vi "Hex string to byte array.vi"(8 "Error In":errorcluster, 11 "Hex string":string) -> (0 "Error Out":errorcluster, 3 "Byte Array":u8[](array[numeric]) format="%02x")   [LabVIEW 2020]
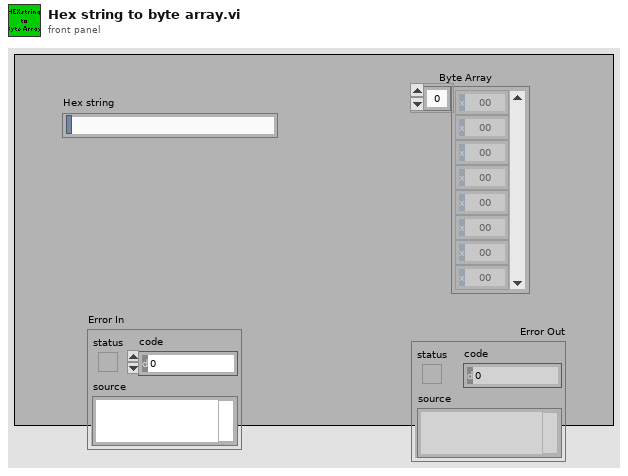
[diagram p1: front panel]
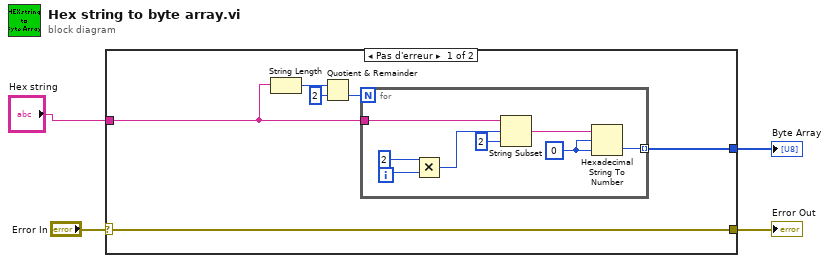
[diagram p0: block diagram]
diagram:
  n1 = case shown="Pas d'erreur" "Error In" {
    selector: "Error In" -> [w10 w19]
    tunnel: [w10 w19] -> w3
    tunnel: "Hex string" -> [w6 _]
    tunnel: [w5 _] -> w2
    frame No Error {
      n2 = String Length(string=w6) -> (length=w7:i32)
      n3 = Quotient & Remainder(x=w7, y=2) -> (floor(x/y)=w9:i32)  [unwired: 1 out]
      n4 = for {
        N: w9 -> [_]
        tunnel: w6 -> [w18]
        tunnel: [w11] -> w5 mode=indexing
        i -> [w17]
        w12 = u8 0 ("default (0 U32)")
        n5 = Multiply(x=2, y=w17) -> (x*y=w15:i32)
        n6 = String Subset(string=w18, offset (0)=w15, length (rest)=2 ("length (rest)")) -> (substring=w13:string)
        n7 = Hexadecimal String To Number(string=w13, offset=w12, default (0uL)=w12) -> (number=w11:u8)  [unwired: 1 out]
      }
    }
    frame Error {
    }
  }
  "Error Out" <- w3
  "Byte Array" <- w2
